vi "GetOneSeries.vi"(8 "error in (no error)":errorcluster, 11 "id":string) -> (0 "error out":errorcluster, 3 "last path":path)   [LabVIEW 2024]
uses:
  <vilib>/addons/_JKI.lib/REST Client/classes/REST Client/REST Client.lvclass
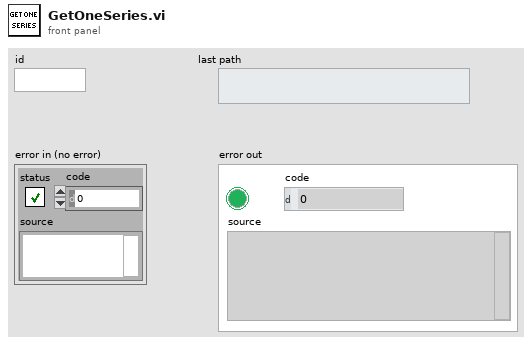
[diagram p1: front panel]
types:
  T1 = typedef "series.reply.ctl" = cluster{"code":i32, "status":string, "etag":string, "data":cluster{"offset":i32, "limit":i32, "total":i32, "count":i32, "results":T2[]}}
  T2 = typedef "series--cluster.ctl" = cluster{"id":i32, "title":string, "description":string, "resourceURI":string, "urls":cluster{"type":string, "url":string}[], "startYear":i32, "endYear":i32, "rating":string, "type":string, "modified":variant, "thumbnail":cluster{"path":string, "extension":string}, "creators":cluster{"available":i32, "returned":i32, "collectionURI":string, "items":cluster{"resourceURI":string, "name":string, "role":string}[]}, "comics":cluster{"available":i32, "returned":i32, "collectionURI":string, "items":cluster{"resourceURI":string, "name":string}[]}, "characters":cluster{"available":i32, "returned":i32, "collectionURI":string, "items":cluster{"resourceURI":string, "name":string}[]}, "stories":cluster{"available":i32, "returned":i32, "collectionURI":string, "items":cluster{"resourceURI":string, "name":string, "type":string}[]}, "events":cluster{"available":i32, "returned":i32, "collectionURI":string, "items":cluster{"resourceURI":string, "name":string}[]}, "next":variant, "previous":variant, "tags":string[]}
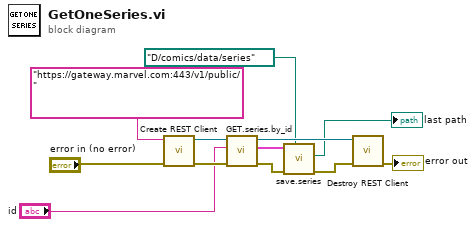
[diagram p0: block diagram]
diagram:
  n1 = call <vilib>:"Create REST Client.vi"("error in (no error)"="error in (no error)", "Base URL"="https://gateway.marvel.com:443/v1/public/") -> ("error out"=w10:errorcluster, "REST Client out"=w11:refnum<class "REST Client.lvclass">)  [unwired: 8 in]
  n2 = call "GET.series.by_id.vi"("error in (no error)"=w10, "id"="id", "REST Client in"=w11) -> ("error out"=w8:errorcluster, "data"=w7:T1, "REST Client out"=w6:refnum<class "REST Client.lvclass">)  [unwired: 6 in]
  n3 = call "save.series.vi"("file (use dialog)"=path "D:/comics/data/series", "error in"=w8, "data"=w7) -> ("error out"=w5:errorcluster, "last path"=→"last path":path)  [unwired: 7 in]
  n4 = call-dynamic "Destroy REST Client.vi"("error in (no error)"=w5, "REST Client in"=w6) -> ("error out"=→"error out":errorcluster)  [unwired: 9 in]
